vi "Settings Dialog.vi"(8 "error in (no error)":errorcluster, 10 "System Control Queue":refnum<queue>, 11 "Plugin Settings":T6={"Acquisition Configuration"={"Query rate (sec)"=1.0}, "Instrument Configuration"={"Device"="", "Firmware Version"=""}, "Logging Configuration"={"Log Directory"=path "", "Log File Format"=enum."Spreadsheet (CSV)", "Log File Name Prefix"="experiment_", "Logging Start Mode"=enum."Manual Start", "Logging Stop Mode"=enum."Log Continuously", "Log Interval (Seconds)"=0.001}, "Connection Info"={"VISA Resource"="", "Address"=1}} {"Connection Info"."Address" min=1; "Logging Configuration"."Log Interval (Seconds)" min=0.0010000000474974513; "Acquisition Configuration"."Query rate (sec)" min=1.0 step=0.1}) -> (0 "error out":errorcluster, 2 "Cancelled?":bool, 3 "Plugin Settings out":T6={"Acquisition Configuration"={"Query rate (sec)"=1.0}, "Instrument Configuration"={"Device"="", "Firmware Version"=""}, "Logging Configuration"={"Log Directory"=path "", "Log File Format"=enum."Spreadsheet (CSV)", "Log File Name Prefix"="experiment_", "Logging Start Mode"=enum."Manual Start", "Logging Stop Mode"=enum."Log Continuously", "Log Interval (Seconds)"=0.001}, "Connection Info"={"VISA Resource"="", "Address"=1}} {"Connection Info"."Address" min=1; "Logging Configuration"."Log Interval (Seconds)" min=0.0010000000474974513; "Acquisition Configuration"."Query rate (sec)" min=1.0 step=0.1})   [LabVIEW 2020, in "plugin_flodx_pressure.lvlib" / "plugin.lvlib"]
doc: "Opens a dialog to get the inlet-outlet port pairings for the pump."
uses:
  plugin.lvlib
  settings.ctl
  <userlib>/RxnRover/PluginCore/src/process loops/Acquisition/Acquisition Config.ctl
  Instrument Manager/Instrument Config.ctl
  <userlib>/RxnRover/PluginCore/src/process loops/Logging/loop/Logging Config.ctl
  <userlib>/RxnRover/PluginCore/src/process loops/Logging/log formats/Supported Log File Formats.ctl
  <userlib>/RxnRover/PluginCore/src/process loops/Logging/logger/Logging Start Mode.ctl
  <userlib>/RxnRover/PluginCore/src/process loops/Logging/logger/Logging Stop Mode.ctl
  Instrument Manager/connection_info/Connection Info.ctl
  <userlib>/RxnRover/PluginCore/src/support/Message Queue/Message Cluster.ctl
  <userlib>/RxnRover/PluginCore/src/process loops/Acquisition/Acquisition.lvlib
  <userlib>/RxnRover/PluginCore/src/process loops/Logging/Logging.lvlib
  Instrument Manager/Instrument Manager.lvlib
  <userlib>/RxnRover/PluginCore/src/support/Message Queue/Message Queue.lvlib
panel:
  in  "Logging Configuration":T1={"Log Directory"=path "", "Log File Format"=enum."Spreadsheet (CSV)", "Log File Name Prefix"="experiment_", "Logging Start Mode"=enum."Manual Start", "Logging Stop Mode"=enum."Log Continuously", "Log Interval (Seconds)"=1.0} {"Log Interval (Seconds)" min=1.0}
  in  "Acquisition Configuration":T5={"Query rate (sec)"=1.0} {"Query rate (sec)" min=1.0 step=0.1}
  in  "Save and Quit Btn":bool
  in  "Cancel Btn":bool
  in  "Reset to Defaults Btn":bool
  in  "Save Changes Btn":bool
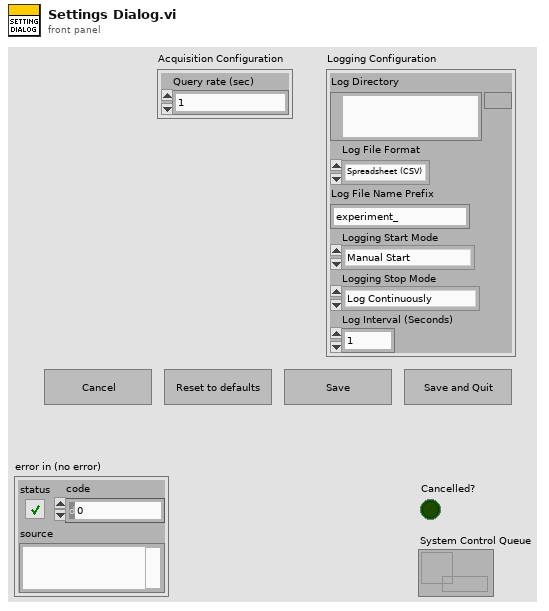
[diagram p1: front panel]
types:
  T1 = typedef "RxnRover_Plugin_Core.lvlib/Logging.lvlib/Logging Config.ctl" = cluster{"Log Directory":path, "Log File Format":T2, "Log File Name Prefix":string, "Logging Start Mode":T3, "Logging Stop Mode":T4, "Log Interval (Seconds)":dbl}
  T2 = typedef "RxnRover_Plugin_Core.lvlib/Logging.lvlib/Supported Log File Formats.ctl" = enum16{"Spreadsheet (CSV)"}
  T3 = typedef "RxnRover_Plugin_Core.lvlib/Logging.lvlib/Logging Start Mode.ctl" = enum16{"Manual Start", "Log While Running"}
  T4 = typedef "RxnRover_Plugin_Core.lvlib/Logging.lvlib/Logging Stop Mode.ctl" = enum16{"Log Continuously", "Log While Running"}
  T5 = typedef "RxnRover_Plugin_Core.lvlib/Acquisition.lvlib/Acquisition Config.ctl" = cluster{"Query rate (sec)":dbl}
  T6 = typedef "plugin_flodx_pressure.lvlib/plugin.lvlib/settings.ctl" = cluster{"Acquisition Configuration":T5, "Instrument Configuration":T7, "Logging Configuration":T1, "Connection Info":T8}
  T7 = typedef "plugin_flodx_pressure.lvlib/plugin.lvlib/Instrument Manager.lvlib/Instrument Config.ctl" = cluster{"Device":string, "Firmware Version":string}
  T8 = typedef "plugin_flodx_pressure.lvlib/plugin.lvlib/Instrument Manager.lvlib/Connection Info.ctl" = cluster{"VISA Resource":refnum<visa-resource-name>, "Address":u8}
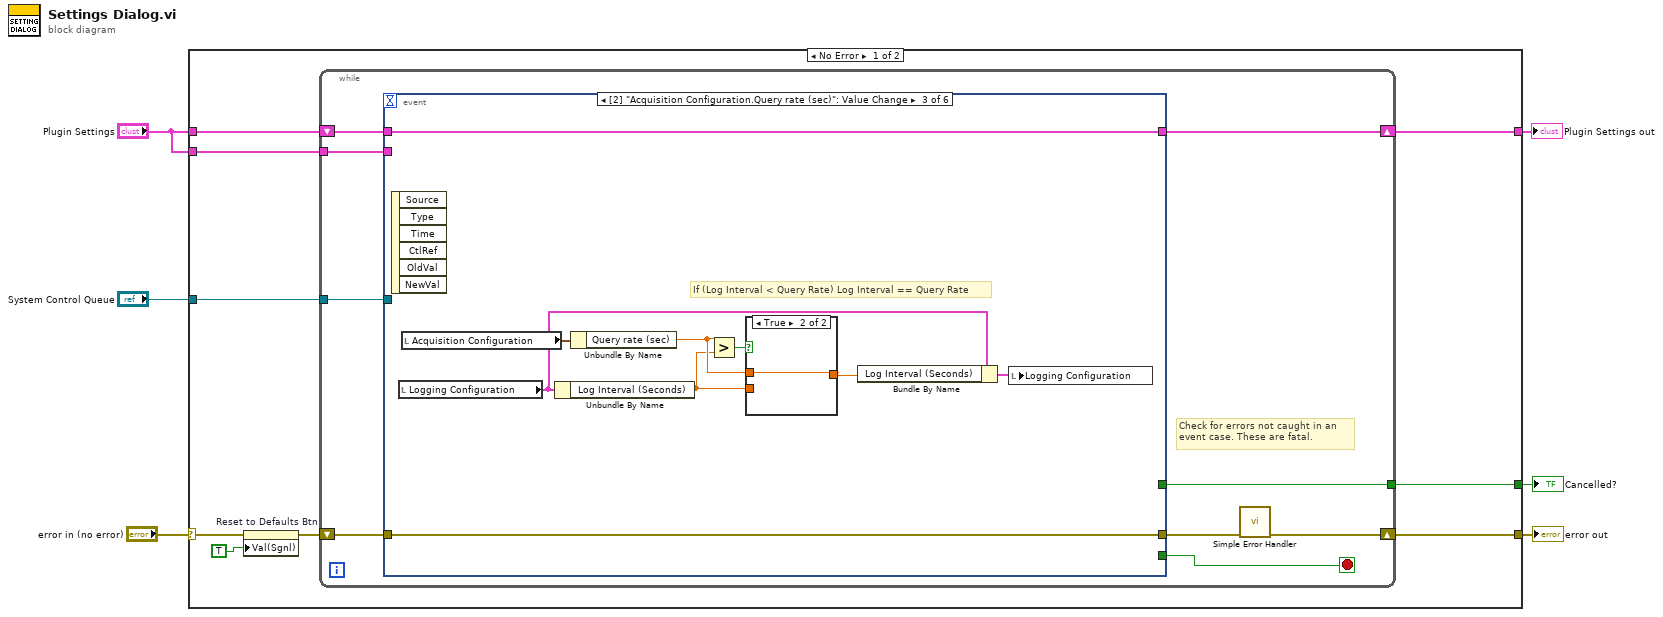
[diagram p0: block diagram]
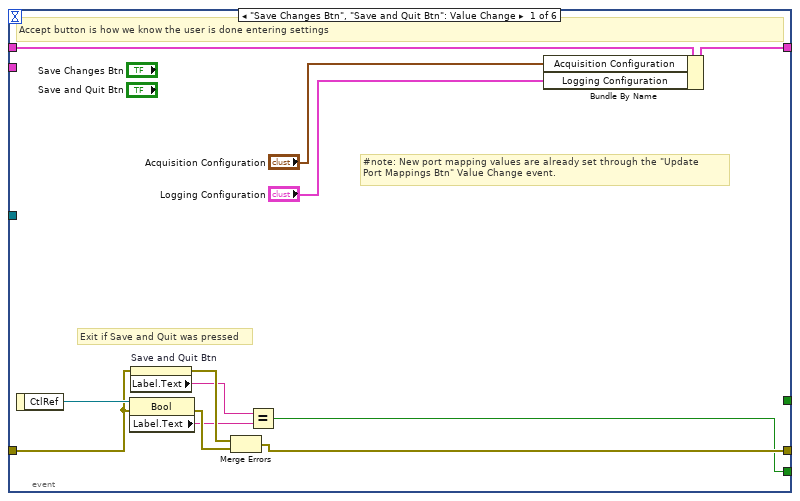
[diagram p2: hidden frame]
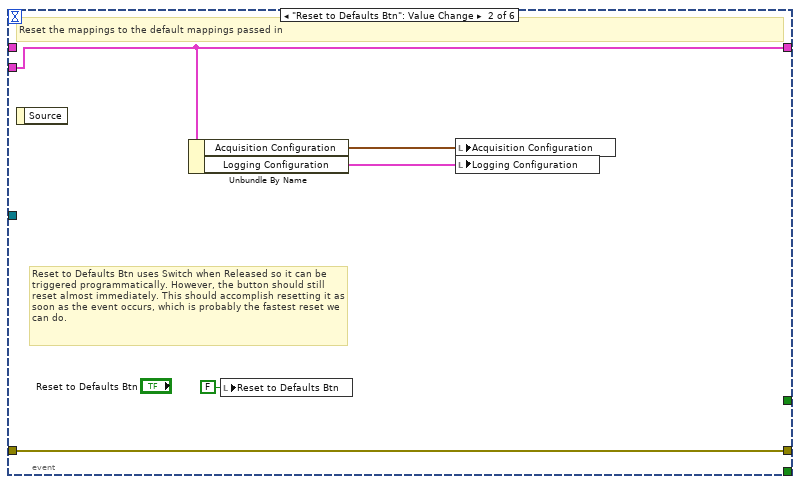
[diagram p3: hidden frame]
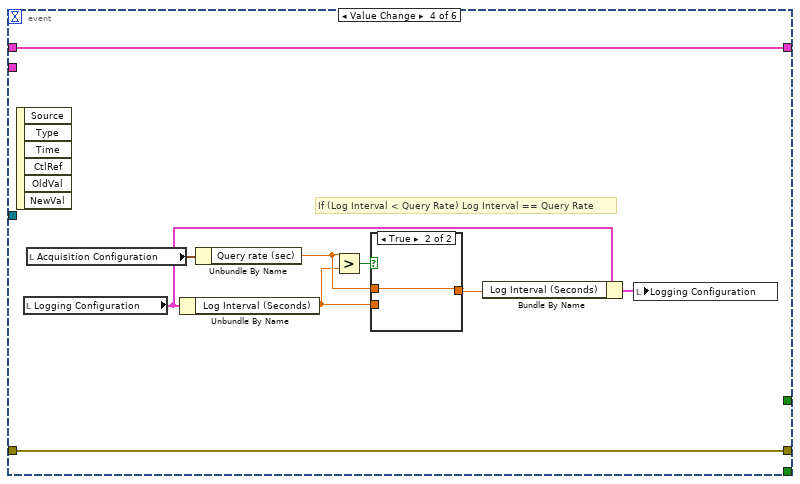
[diagram p5: hidden frame]
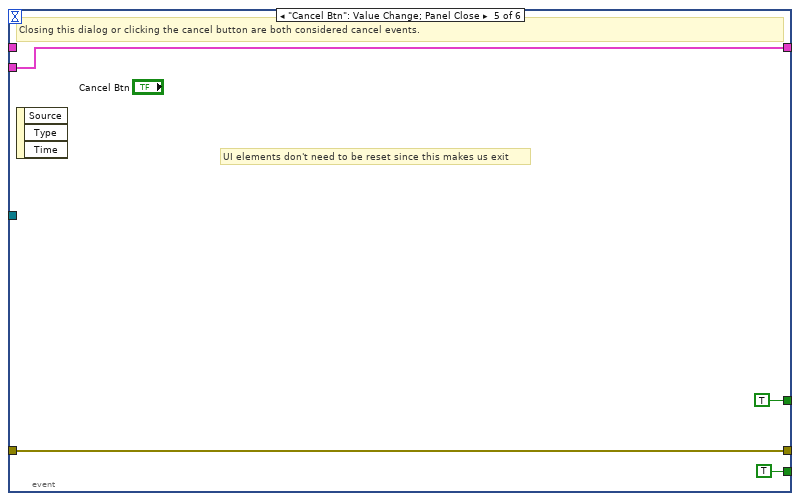
[diagram p7: hidden frame]
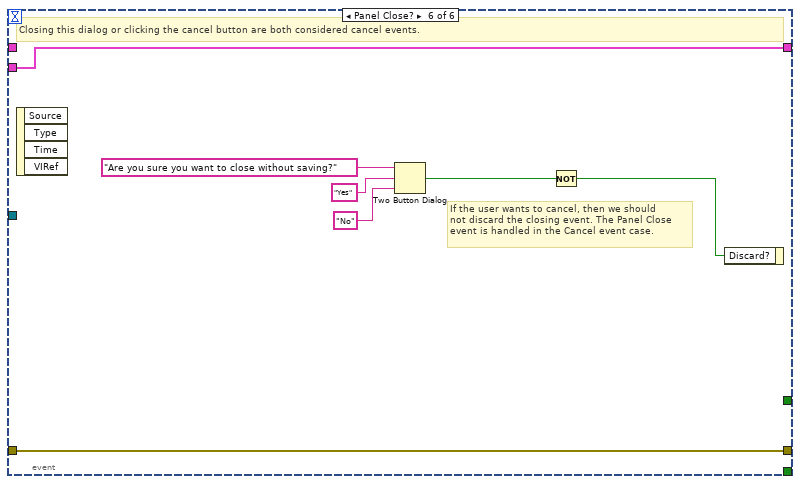
[diagram p8: hidden frame]
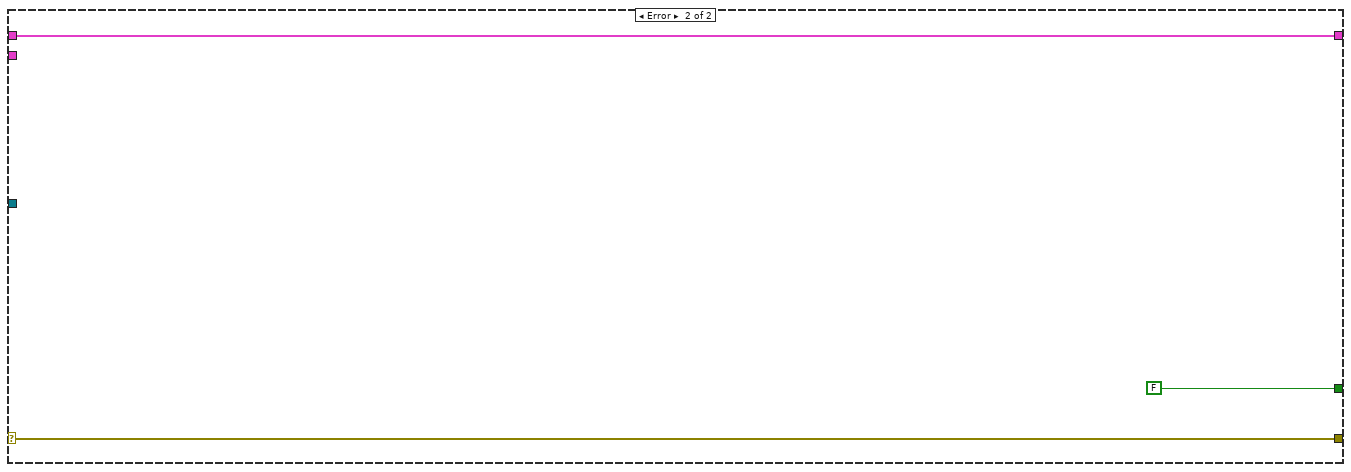
[diagram p9: hidden frame]
diagram:
  n1 = case shown="No Error" "error in (no error)" {
    selector: "error in (no error)" -> [w11 w77]
    tunnel: [w13 w77] -> w5
    tunnel: "Plugin Settings" -> [w15 w75]
    tunnel: [w14 w75] -> w2
    tunnel: [w12 FALSE] -> w4
    tunnel: "Plugin Settings" -> [w10 _]
    tunnel: "System Control Queue" -> [w7 _]
    frame No Error {
      n2 = property on="Reset to Defaults Btn" class="Bool (strict)"(error in=w11, "Val(Sgnl)"=TRUE) -> (error out=w9:errorcluster)  [unwired: 1 in, 1 out]
      n3 = while {
        shift-right: [w21] -> w14
        shift-left: w15 -> [w24]
        shift-right: [w17] -> w13
        shift-left: w9 -> [w23]
        tunnel: w10 -> [w19]
        tunnel: [w18] -> w12
        tunnel: w7 -> [w16]
        stop <- w20 stop-if-true
        # "Check for errors not caught in an\nevent case. These are fatal."
        n4 = event shown="[2] \"Acquisition Configuration.Query rate (sec)\": Value Change" {
          selector: _ -> [_ _ _ _ _ _]
          dyn-events: _ -> [_ _ _ _ _ _]
          timeout: _ -> [_ _ _ _ _ _]
          tunnel: w24 -> [w36 _ w45 w56 _ _]
          tunnel: w23 -> [w34 w41 w48 w59 w66 w73]
          tunnel: [w31 w41 w48 w59 w66 w73] -> w22
          tunnel: [w27 w40 w45 w56 w67 w74] -> w21
          tunnel: [w28 _ _ _ TRUE _] -> w20
          tunnel: w19 -> [_ w40 _ _ w67 w74]
          tunnel: [_ _ _ _ TRUE _] -> w18
          tunnel: w16 -> [_ _ _ _ _ _]
          event "Save Changes Btn", "Save and Quit Btn": Value Change {
            # "#note: New port mapping values are already set through the \"Update\nPort Mappings Btn\" Value Change event."
            # "Exit if Save and Quit was pressed"
            # "Accept button is how we know the user is done entering settings"
            n5 = event-data() -> ("CtlRef"=w35:refnum<vi>)  [unwired: 1 in]
            n6 = property class="Bool"(reference=w35, error in=w34) -> (error out=w33:errorcluster, "Label.Text"=w29:string)  [unwired: 1 out]
            n7 = property on="Save and Quit Btn" class="Bool"(error in=w34) -> (error out=w32:errorcluster, "Label.Text"=w30:string)  [unwired: 1 in, 1 out]
            n8 = Merge Errors(w32, w33) -> (w31:errorcluster)
            n9 = Equal?(x=w30, y=w29) -> (x = y?=w28:bool)
            n10 = Bundle By Name(cluster=w36, "Acquisition Configuration"="Acquisition Configuration", "Logging Configuration"="Logging Configuration") -> (w27:T6)
          }
          event "Reset to Defaults Btn": Value Change {
            # "Reset to Defaults Btn uses Switch when Released so it can be triggered programmatically. However, the button should still reset almost immediately. This should accomplish resetting it as soon as the event occurs, which is probably the fastest reset we can do."
            # "Reset the mappings to the default mappings passed in"
            n11 = event-data() -> ()  [unwired: 1 in, 1 out]
            n12 = Unbundle By Name(w40) -> ("Acquisition Configuration"=w39:T5, "Logging Configuration"=w38:T1)
            n13 = local write "Reset to Defaults Btn"(FALSE ("Reset to Defaults Btn")) -> ()
            n14 = local write "Acquisition Configuration"(w39) -> ()
            n15 = local write "Logging Configuration"(w38) -> ()
          }
          event Value Change {
            # "If (Log Interval < Query Rate) Log Interval == Query Rate"
            n16 = event-data() -> ()  [unwired: 1 in, 6 out]
            n17 = local read "Logging Configuration"() -> (w42:T1)
            n18 = local read "Acquisition Configuration"() -> (w47:T5)
            n19 = Unbundle By Name(w42) -> ("Log Interval (Seconds)"=w46:dbl)
            n20 = Unbundle By Name(w47) -> ("Query rate (sec)"=w49:dbl)
            n21 = Greater?(x=w49, y=w46) -> (0:w50:bool)
            n22 = case shown="True" w50 {
              tunnel: w49 -> [_ w52]
              tunnel: w46 -> [w51 _]
              tunnel: [w51 w52] -> w44
              frame False {
              }
              frame True {
              }
            }
            n23 = Bundle By Name(cluster=w42, "Log Interval (Seconds)"=w44) -> (w43:T1)
            n24 = local write "Logging Configuration"(w43) -> ()
          }
          event Value Change {
            # "If (Log Interval < Query Rate) Log Interval == Query Rate"
            n25 = event-data() -> ()  [unwired: 1 in, 6 out]
            n26 = local read "Logging Configuration"() -> (w53:T1)
            n27 = local read "Acquisition Configuration"() -> (w58:T5)
            n28 = Unbundle By Name(w53) -> ("Log Interval (Seconds)"=w57:dbl)
            n29 = Unbundle By Name(w58) -> ("Query rate (sec)"=w60:dbl)
            n30 = Greater?(x=w60, y=w57) -> (0:w61:bool)
            n31 = case shown="True" w61 {
              tunnel: w60 -> [_ w63]
              tunnel: w57 -> [w62 _]
              tunnel: [w62 w63] -> w55
              frame False {
              }
              frame True {
              }
            }
            n32 = Bundle By Name(cluster=w53, "Log Interval (Seconds)"=w55) -> (w54:T1)
            n33 = local write "Logging Configuration"(w54) -> ()
          }
          event "Cancel Btn": Value Change; Panel Close {
            # "UI elements don't need to be reset since this makes us exit"
            # "Closing this dialog or clicking the cancel button are both considered cancel events."
            n34 = event-data() -> ()  [unwired: 1 in, 3 out]
          }
          event Panel Close? {
            # "If the user wants to cancel, then we should\nnot discard the closing event. The Panel Close\nevent is handled in the Cancel event case."
            # "Closing this dialog or clicking the cancel button are both considered cancel events."
            n35 = event-data() -> ()  [unwired: 1 in, 4 out]
            n36 = Two Button Dialog(message="Are you sure you want to close without saving?", 1:"No" ("F button name (\"Cancel\")"), 2:"Yes" ("T button name (\"OK\")")) -> (T button?=w69:bool)
            n37 = Not(x=w69) -> (.not. x?=w68:bool)
            n38 = event-data("Discard?"=w68) -> ()  [unwired: 1 in, 1 out]
          }
        }
        n39 = call <vilib>:"Simple Error Handler.vi"("error in (no error)"=w22) -> ("error out"=w17:errorcluster)  [unwired: 4 in, 4 out]
      }
    }
    frame Error {
    }
  }
  "error out" <- w5
  "Cancelled?" <- w4
  "Plugin Settings out" <- w2
